vi "MB_TCP_70H16_p.vi"(6 "N":i32, 9 "timeouts":T1={"conn_timeout"=1000, "reconn_timeout"=3000, "N attempt max"=3, "t_reset_TTL"=120000, "write_timeout"=10, "read_timeout"=500, "period"=100} {"t_reset_TTL" min=10 max=240000 step=1; "period" min=10 max=100000 step=1; "read_timeout" min=10 max=60000 step=1; "write_timeout" min=1 max=60000 step=1; "N attempt max" min=1 max=5 step=1; "reconn_timeout" min=10 max=240000 step=1; "conn_timeout" min=10 max=240000}, 10 "write enable":bool=TRUE, 11 "stop":bool) -> (0 "error out":errorcluster, 2 "errors":u32, 3 "Z3":u32)   [LabVIEW 2019]
uses:
  NI_modbus_upd/NI_modbus_upd.lvlib
  NI_modbus_upd.llb/MB Modbus Command.ctl
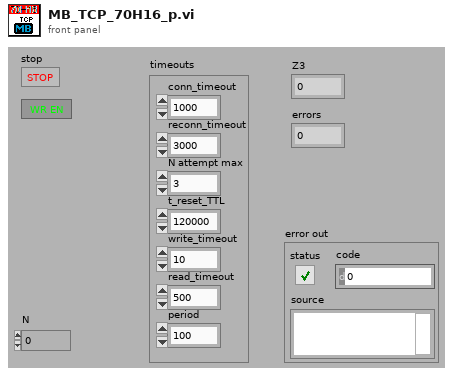
[diagram p1: front panel]
types:
  T1 = cluster{"conn_timeout":i32, "reconn_timeout":u32, "N attempt max":i32, "t_reset_TTL":u32, "write_timeout":i32, "read_timeout":i32, "period":u32}
  T2 = enum16{"Init", "Read", "Read inputs", "Read outputs", "Write", "Write inputs"}
  T3 = enum16{"DI", "DO to write", "DO", "AI", "AO to write", "AO", "DI AI", "DI AO", "DO AI", "DO AO"}
  T4 = enum16{"Start", "Connect", "Write enable", "IP address", "Errors"}
  T5 = typedef "MB Modbus Command.ctl" = cluster{"Function Code":u8, "Starting Address":u16, "Quantity":u16, "Data":u16[], "Discrete":bool[]}
  T6 = cluster{"Transaction ID":u16, "Protocol ID":u16, "Length":u16, "Unit ID":u8}
  T7 = cluster{"Remote IP Address":string, "Remote Port":u16}
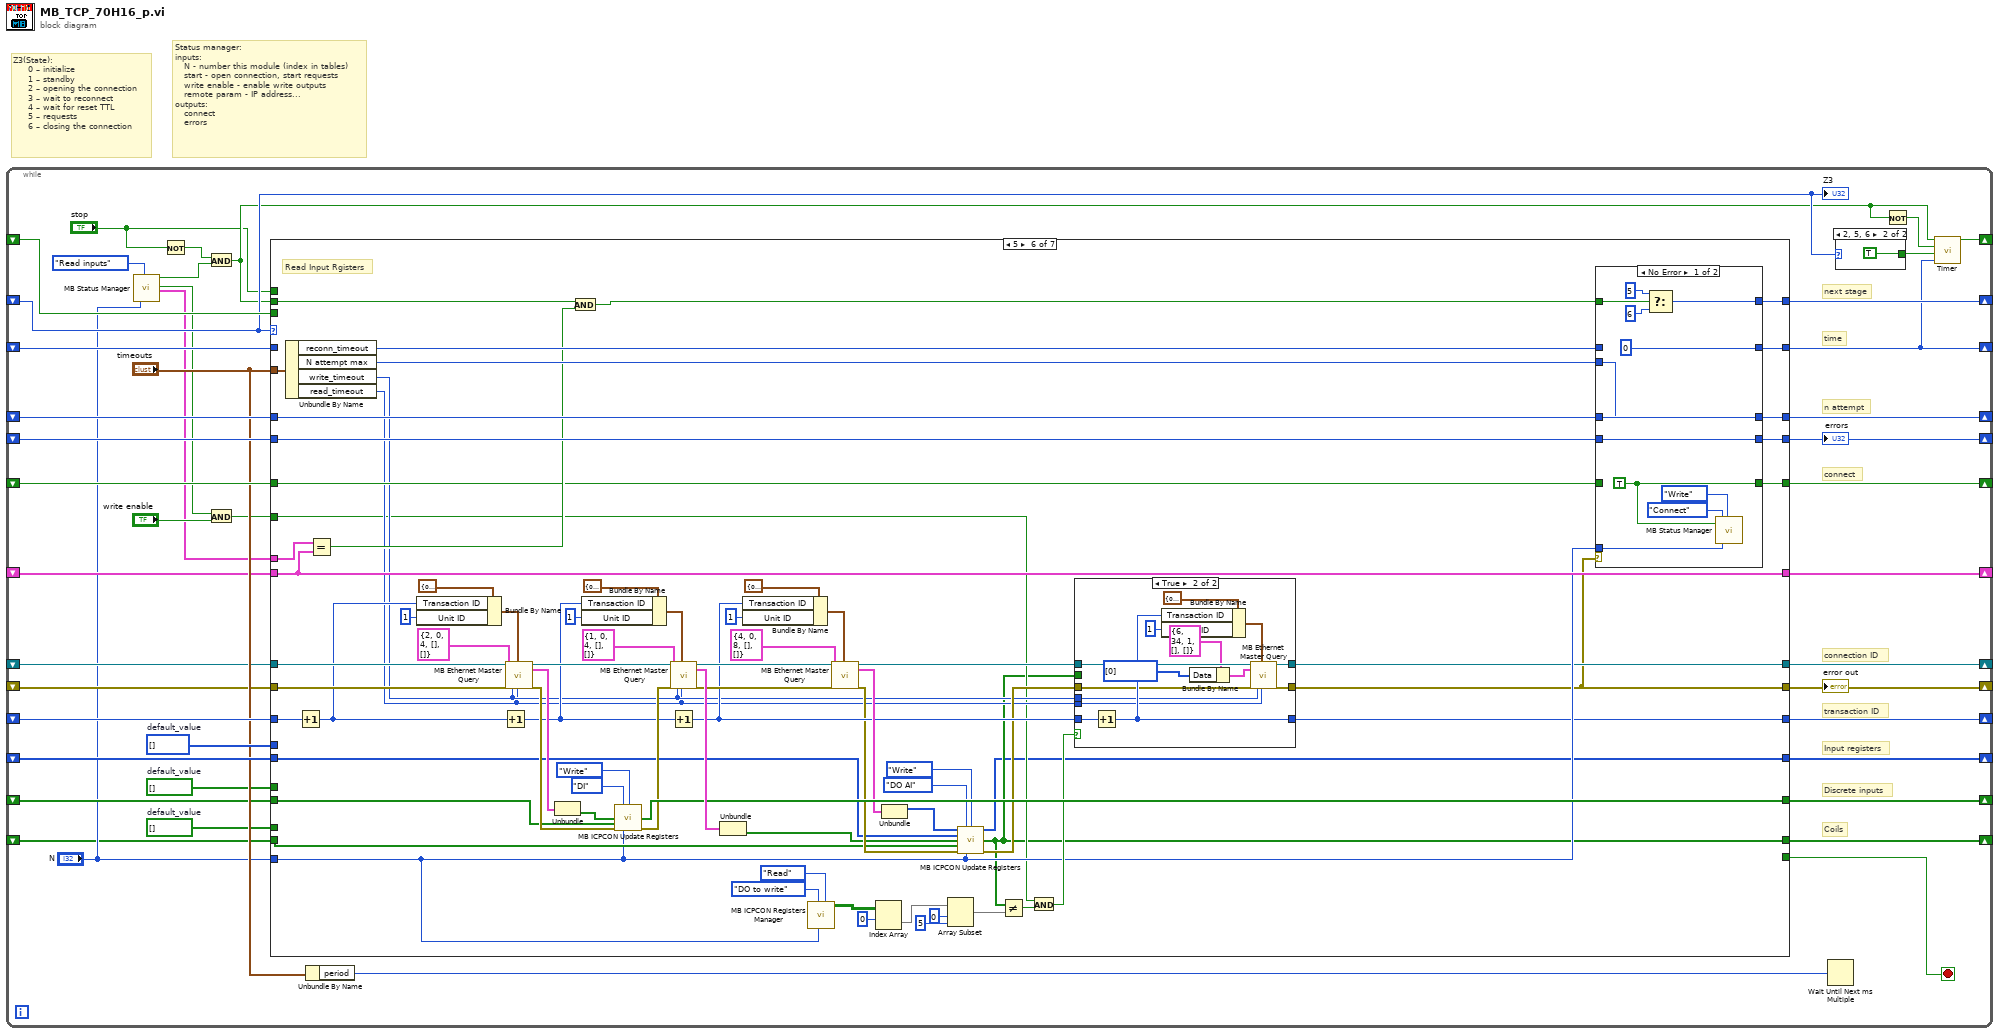
[diagram p0: block diagram]
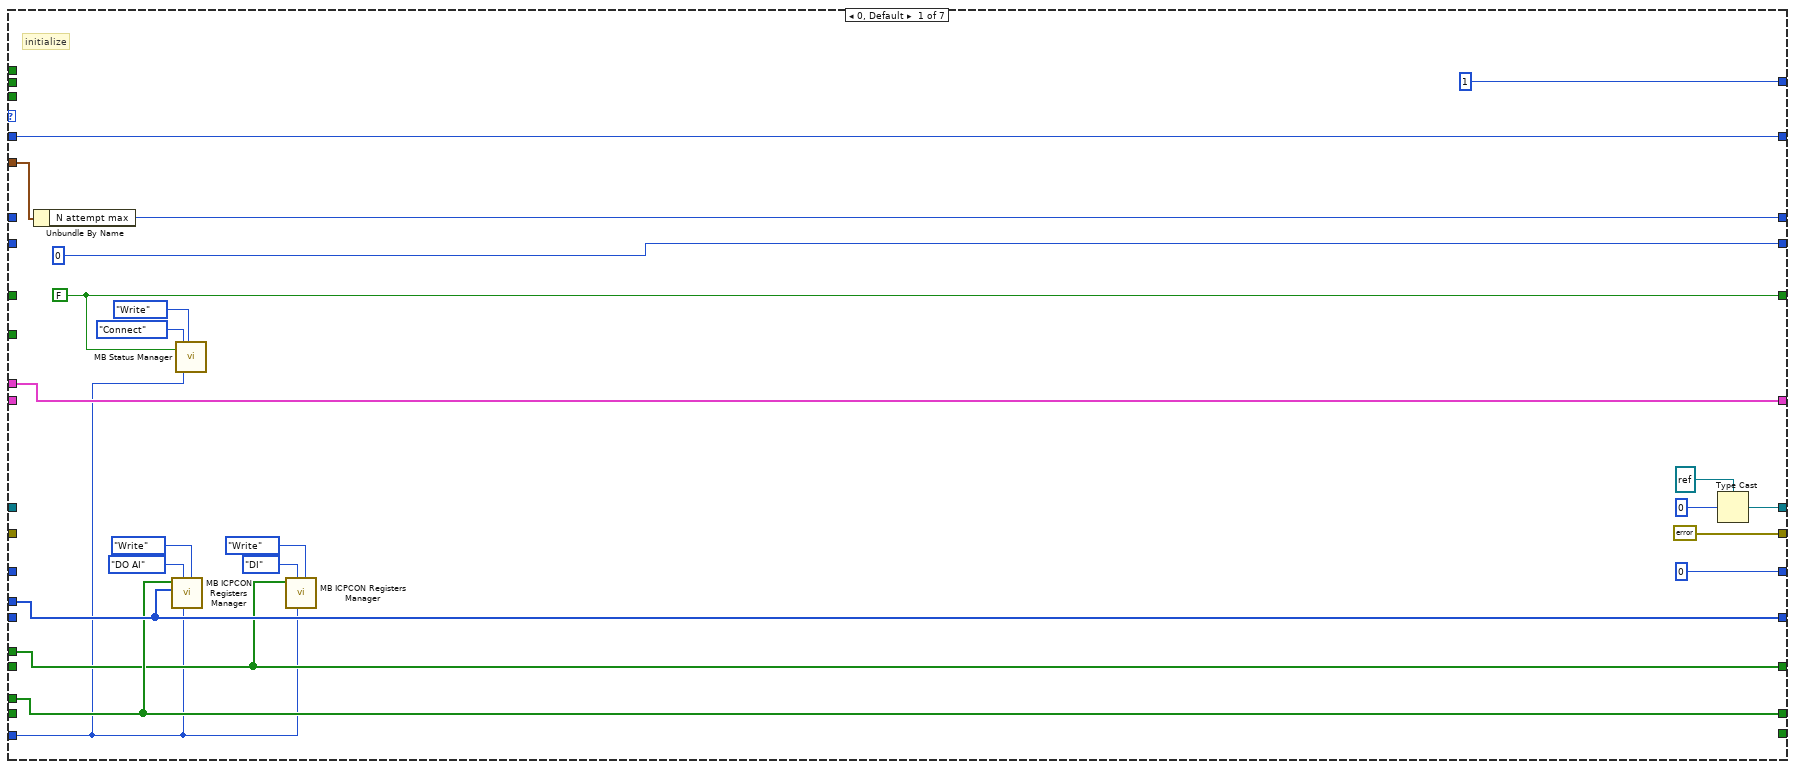
[diagram p2: hidden frame]
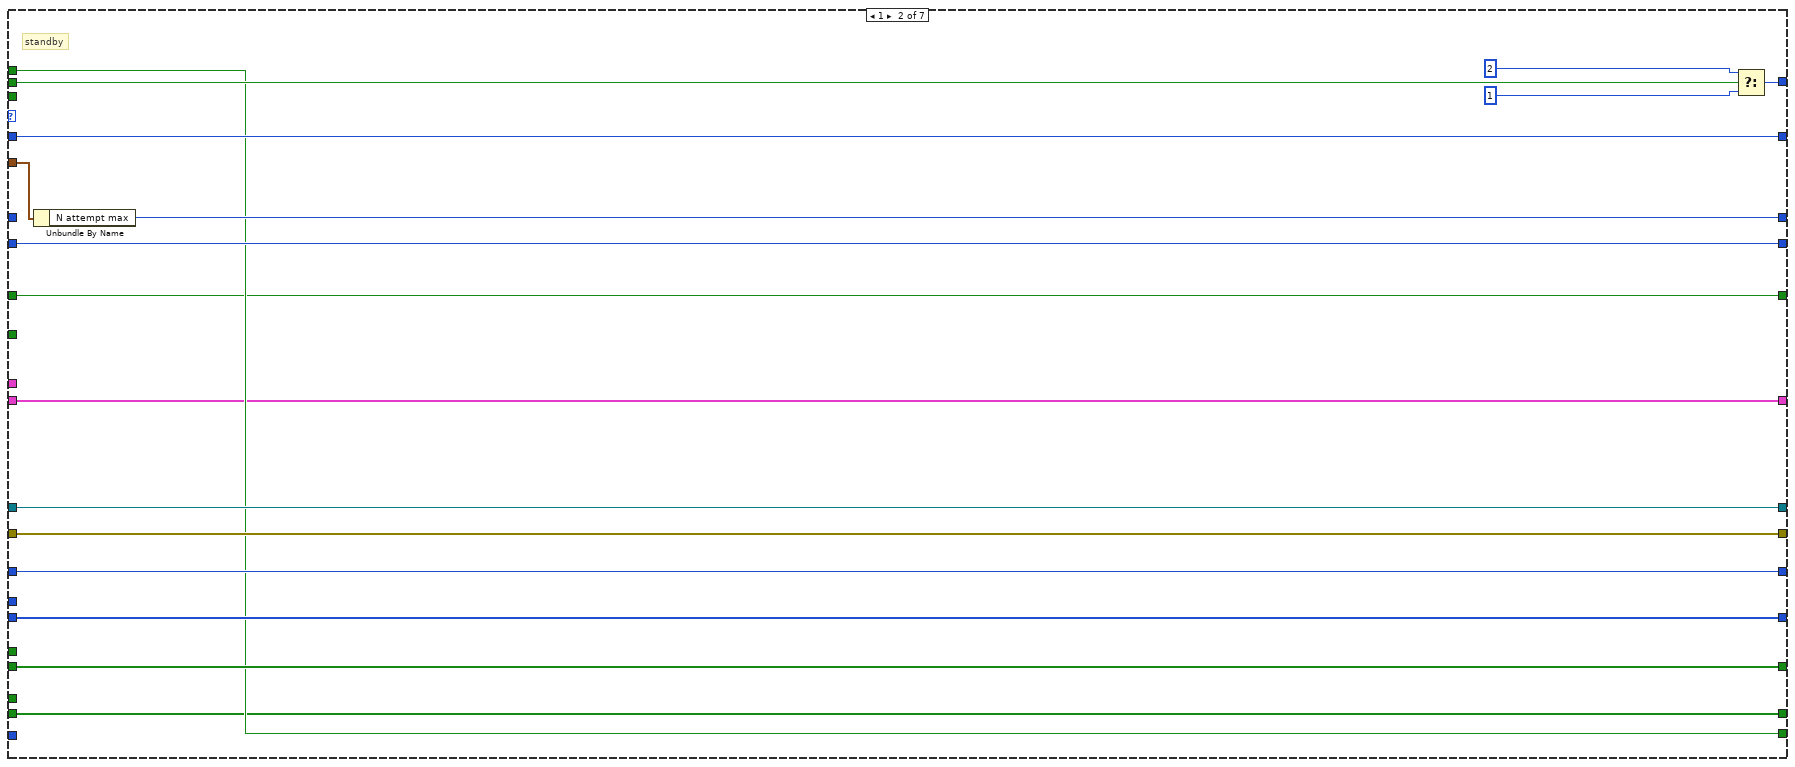
[diagram p3: hidden frame]
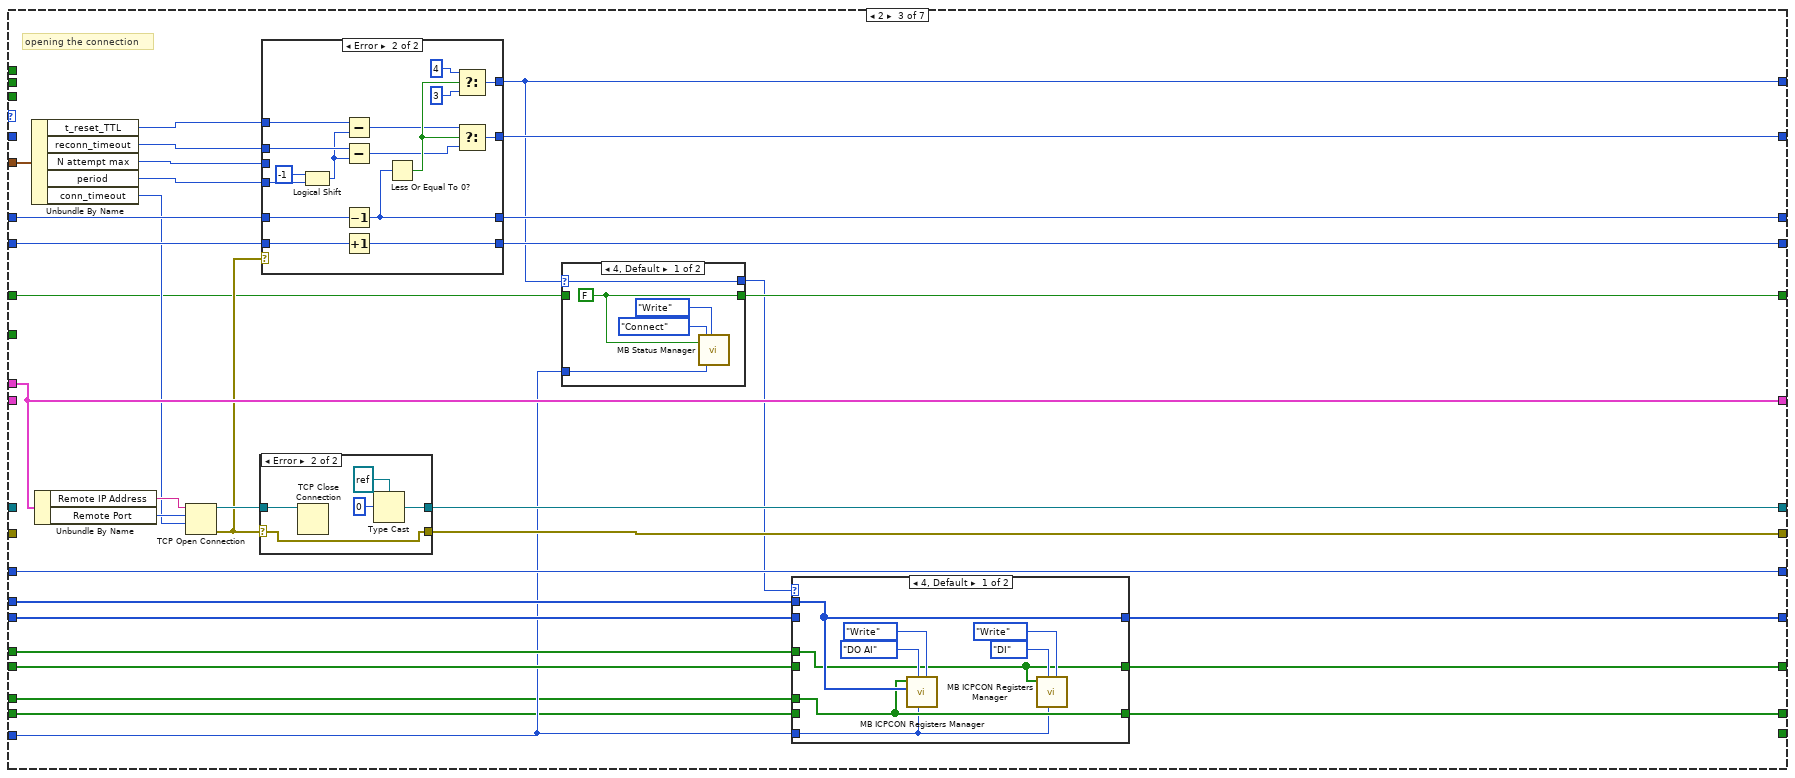
[diagram p4: hidden frame]
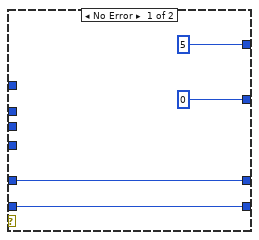
[diagram p8: hidden frame]
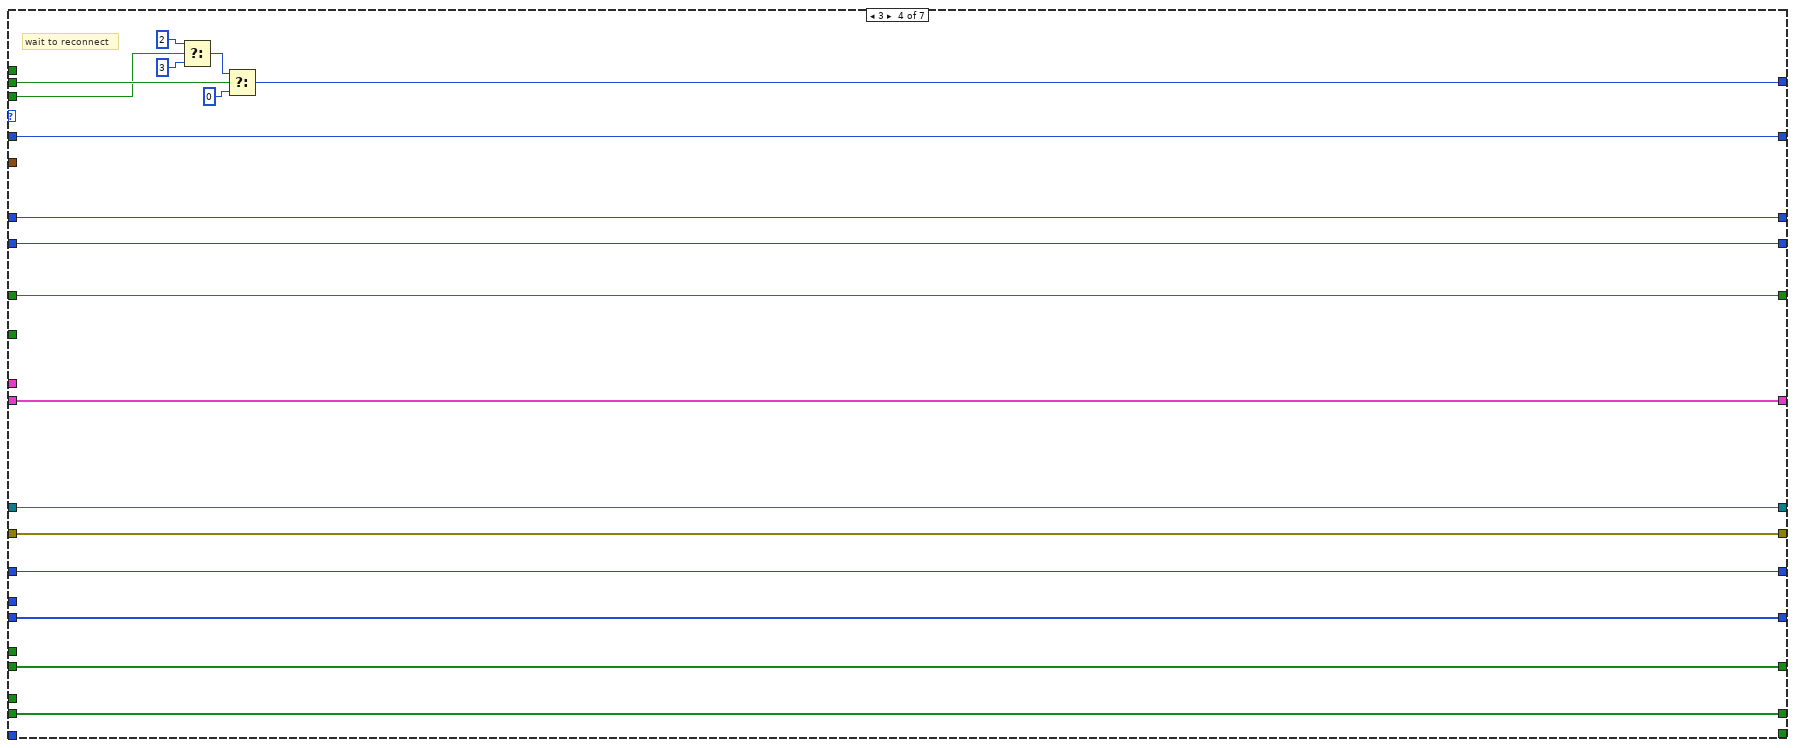
[diagram p9: hidden frame]
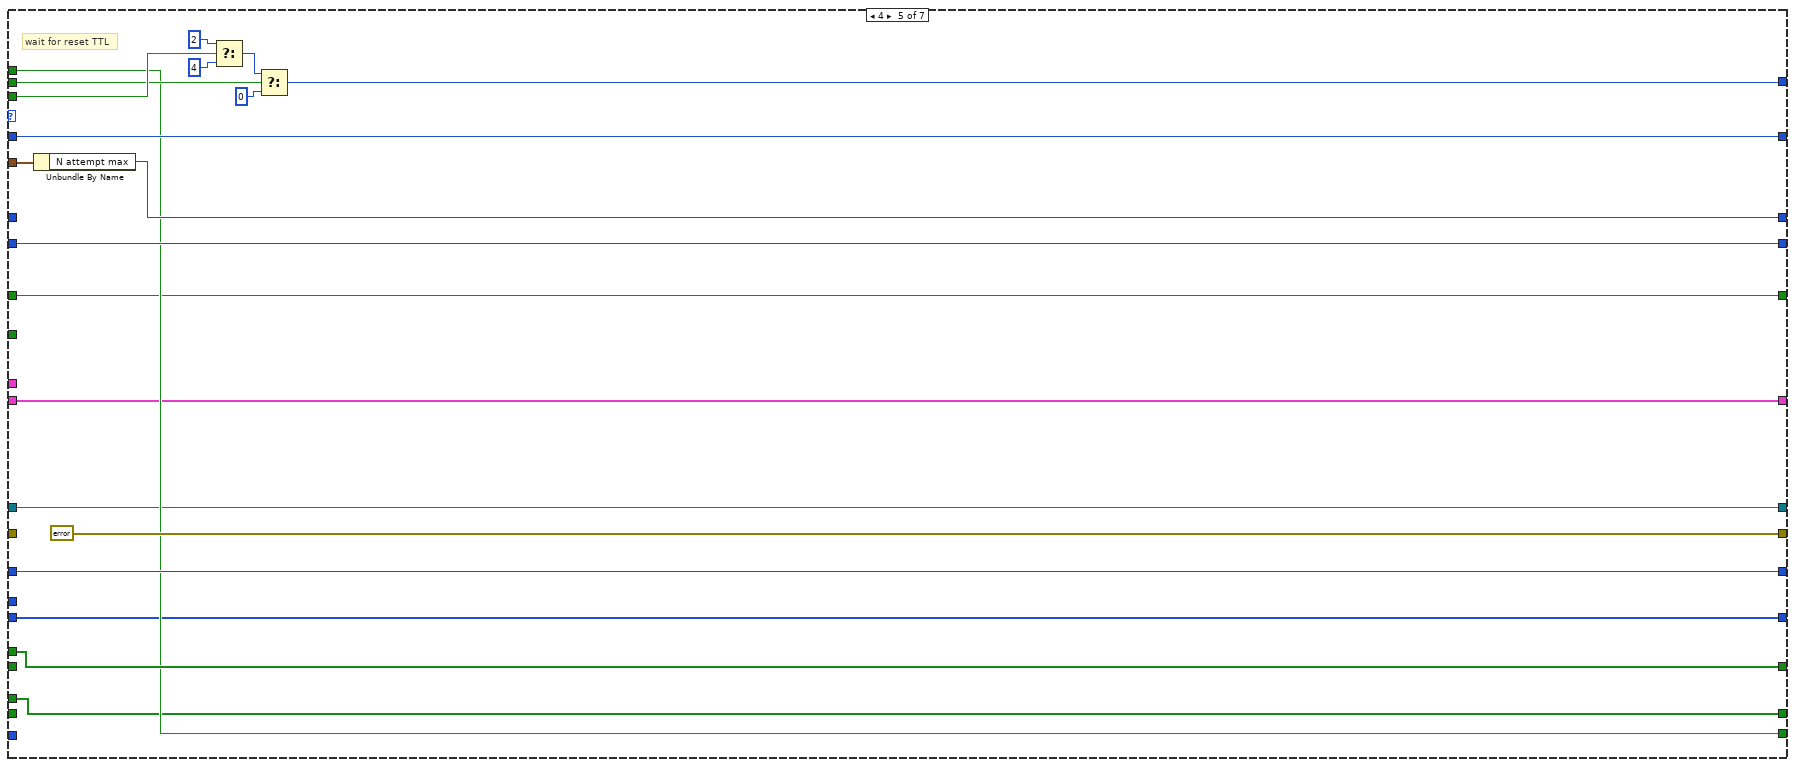
[diagram p10: hidden frame]
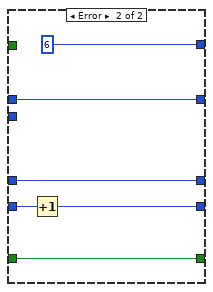
[diagram p12: hidden frame]
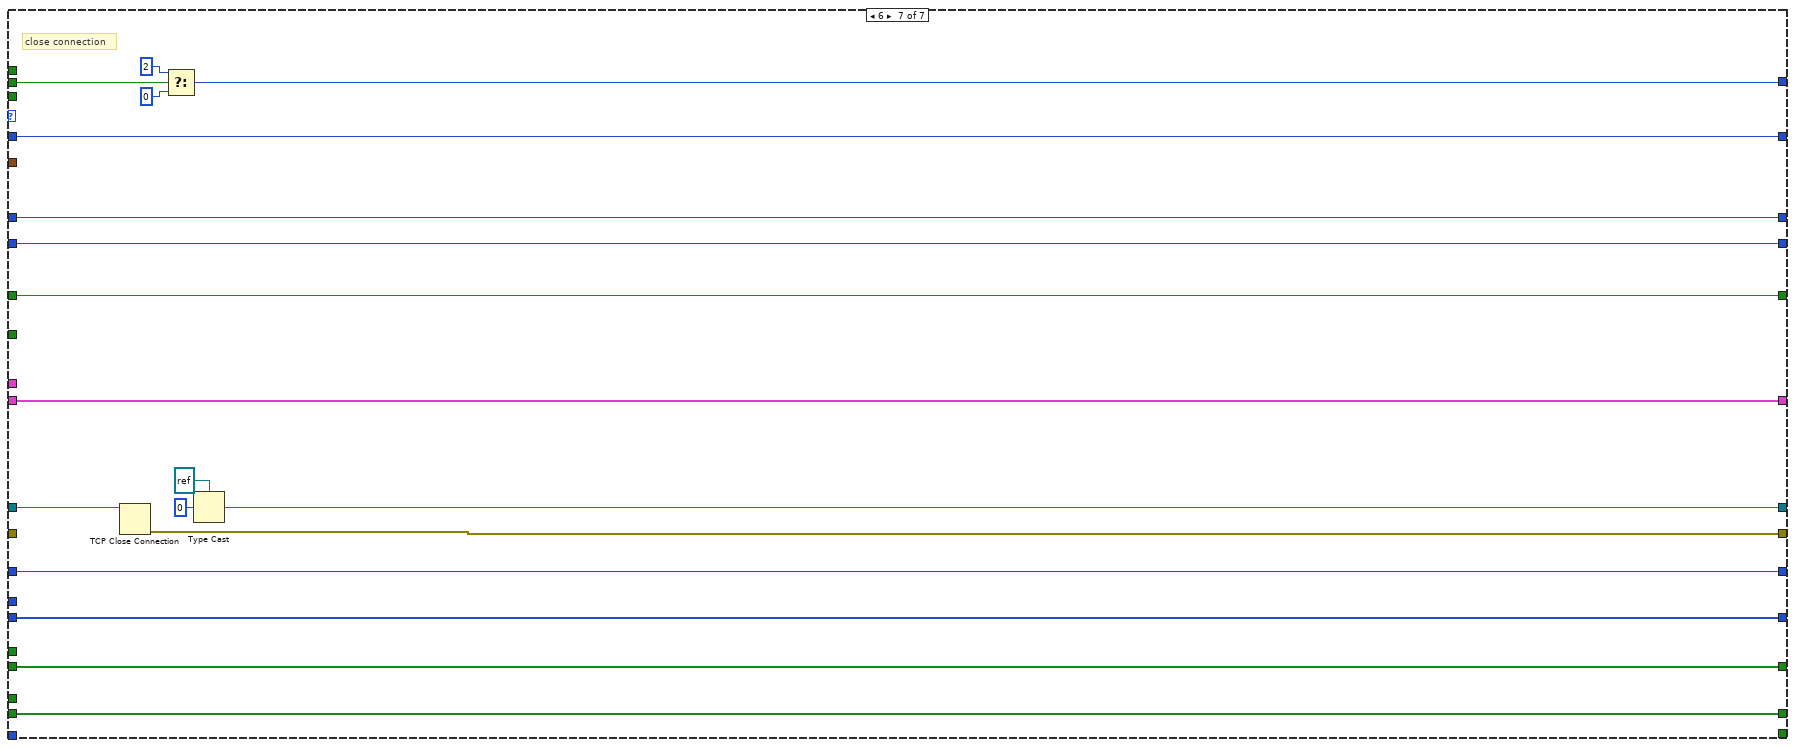
[diagram p13: hidden frame]
diagram:
  # "Status manager:\ninputs:\n   N - number this module (index in tables)\n   start - open connection, start requests\n   write enable - enable write outputs\n   remote param - IP address...\noutputs:\n   connect\n   errors"
  # "Z3(State):\n     0 – initialize \n     1 – standby\n     2 – opening the connection\n     3 – wait to reconnect\n     4 – wait for reset TTL\n     5 – requests\n     6 – closing the connection"
  n1 = while {
    shift-right: [w21] -> _
    shift-left: _ -> [w17]
    shift-right: [w20] -> _
    shift-left: _ -> [w43]
    shift-right: [w42] -> _
    shift-left: _ -> [w40]
    shift-right: [w41] -> _
    shift-left: _ -> [w39]
    shift-right: [w38] -> _
    shift-left: _ -> [w37]
    shift-right: [w36] -> _
    shift-left: _ -> [w22]
    shift-right: [w35] -> _
    shift-left: _ -> [w23]
    shift-right: [w34] -> _
    shift-left: _ -> [w33]
    shift-right: [w32] -> _
    shift-left: _ -> [w31]
    shift-right: [w25] -> _
    shift-left: _ -> [w24]
    shift-right: [w19] -> _
    shift-left: _ -> [w18]
    shift-right: [w10] -> _
    shift-left: _ -> [w9]
    shift-right: [w2] -> _
    shift-left: _ -> [w4]
    stop <- w13 stop-if-true
    w3 = bool[] []  # default_value
    w26 = bool[] []  # default_value
    w30 = u16[] []  # default_value
    # "Coils"
    # "Discrete inputs"
    # "Input registers"
    # "connect"
    # "connection ID"
    # "transaction ID"
    # "n attempt"
    # "time"
    # "next stage"
    n2 = call "MB Status Manager.vi"("N"="N", "Function"=T2."Read inputs") -> ("start"=w8:bool, "write enable"=w7:bool, "Remote Param"=w6:T7)  [unwired: 12 in, 3 out]
    n3 = Not(x="stop") -> (.not. x?=w15:bool)
    n4 = And(x=w15, y=w8) -> (x .and. y?=w16:bool)
    n5 = And(x=w7, y="write enable") -> (x .and. y?=w12:bool)
    n6 = case shown="5" w17 {
      tunnel: [w64 w74 w94 w177 w184 w201 w323] -> w36
      tunnel: [errorcluster {"status"=FALSE, "code"=0, "source"=""} ("error out") w73 w92 w176 errorcluster {"status"=FALSE, "code"=0, "source"=""} ("error out") w200 w324] -> w35
      tunnel: w22 -> [_ w74 _ w177 w184 w264 w320]
      tunnel: w23 -> [_ w73 _ w176 _ w263 _]
      tunnel: [w53 w69 w90 w165 w183 w251 w311] -> w38
      tunnel: w37 -> [_ w69 w91 w165 w183 w252 w311]
      tunnel: w6 -> [w56 _ w97 _ _ w258 _]
      tunnel: [w52 w75 w102 w164 w182 w203 w310] -> w32
      tunnel: w31 -> [_ w75 w103 w164 w182 w212 w310]
      tunnel: w33 -> [_ w83 w116 w179 w199 w273 w325]
      tunnel: [u16 0 ("x") w83 w116 w179 w199 w202 w325] -> w34
      tunnel: [w58 w79 w111 w178 w195 w271 w317] -> w42
      tunnel: w40 -> [_ _ w112 w178 _ w271 w317]
      tunnel: [u32 0 ("N attempt max") w82 w114 w175 w198 w270 w322] -> w41
      tunnel: w39 -> [_ w82 w115 w175 w198 w269 w322]
      tunnel: [w60 w81 w108 w174 w197 w266 w321] -> w20
      tunnel: w43 -> [w60 w81 _ w174 w197 _ w321]
      tunnel: "timeouts" -> [w59 w80 w113 _ w196 w272 _]
      tunnel: w16 -> [_ w71 _ w170 w186 w257 w318]
      tunnel: [u32 1 w76 w88 w166 w190 w265 w312] -> w21
      tunnel: w18 -> [_ _ _ w168 w189 _ _]
      tunnel: w30 -> [w52 _ w101 _ _ _ _]
      tunnel: w26 -> [w47 _ w98 _ w187 _ _]
      tunnel: [w47 w72 w99 w167 w187 w241 w315] -> w25
      tunnel: w24 -> [_ w72 w100 w167 _ w214 w315]
      tunnel: "N" -> [w46 _ w89 _ _ w209 _]
      tunnel: "stop" -> [_ w70 _ _ w185 _ _]
      tunnel: [_ w70 _ _ w185 _ _] -> w13
      tunnel: w12 -> [_ _ _ _ _ w205 _]
      tunnel: [w56 w68 w97 w163 w181 w255 w309] -> w10
      tunnel: w9 -> [_ w68 _ w163 w181 w255 w309]
      tunnel: w3 -> [w50 _ w86 _ w180 _ _]
      tunnel: w4 -> [_ w67 w85 w162 _ w210 w308]
      tunnel: [w50 w67 w84 w162 w180 w204 w308] -> w2
      frame 0, Default {
        w53 = FALSE ("connect")
        # "initialize"
        n7 = Unbundle By Name(w59) -> ("N attempt max"=w58:i32)
        n8 = call "MB ICPCON Registers Manager.vi"("Function"=enum16{"Init", "Read", "Write", "Read All"}."Write", "N"=w46, "Table"=T3."DO AI", "Registers In"=w52, "Discrete in"=w50) -> ()  [unwired: 4 in, 3 out]
        n9 = call "MB Status Manager.vi"("connect in"=w53, "Table"=T4."Connect", "N"=w46, "Function"=T2."Write") -> ()  [unwired: 10 in, 6 out]
        n10 = call "MB ICPCON Registers Manager.vi"("Function"=enum16{"Init", "Read", "Write", "Read All"}."Write", "N"=w46, "Table"=T3."DI", "Discrete in"=w47) -> ()  [unwired: 5 in, 3 out]
        n11 = Type Cast(type=refnum<k5> refnum ("connection ID"), x=u32 0) -> (*(type *) &x=w64:refnum<k5>)
      }
      frame 1 {
        # "standby"
        n12 = Unbundle By Name(w80) -> ("N attempt max"=w79:i32)
        n13 = Select(t=u32 2, s=w71, f=u32 1) -> (s? t:f=w76:u32)
      }
      frame 2 {
        # "opening the connection"
        n14 = Unbundle By Name(w113) -> ("t_reset_TTL"=w107:u32, "reconn_timeout"=w109:u32, "N attempt max"=w110:i32, "period"=w104:u32, "conn_timeout"=w96:i32)
        n15 = Unbundle By Name(w97) -> ("Remote IP Address"=w106:string, "Remote Port"=w105:u16)
        n16 = TCP Open Connection(address=w106, remote port or service name=w105, timeout ms (60000)=w96) -> (connection ID=w95:refnum<k5>, error out=w93:errorcluster)  [unwired: 2 in]
        n17 = case shown="Error" w93 {
          selector: w93 -> [w124 w126]
          tunnel: w95 -> [w125 w129]
          tunnel: [w125 w128] -> w94
          tunnel: [w124 w126] -> w92
          frame No Error {
          }
          frame Error {
            n18 = TCP Close Connection(connection ID=w129) -> ()  [unwired: 2 in, 2 out]
            n19 = Type Cast(type=refnum<k5> refnum ("connection ID"), x=u32 0) -> (*(type *) &x=w128:refnum<k5>)
          }
        }
        n20 = case shown="Error" w93 {
          tunnel: w115 -> [w145 w161]
          tunnel: [w145 w160] -> w114
          tunnel: w112 -> [w144 w159]
          tunnel: [w144 w158] -> w111
          tunnel: w110 -> [_ _]
          tunnel: [u32 5 w155] -> w88
          tunnel: w109 -> [_ w154]
          tunnel: [u32 0 w153] -> w108
          tunnel: w107 -> [_ w150]
          tunnel: w104 -> [_ w148]
          frame No Error {
          }
          frame Error {
            n21 = Logical Shift(y=i16 -1, x=w148) -> (x << y=w146:u32)
            n22 = Subtract(x=w150, y=w146) -> (x-y=w149:u32)
            n23 = Subtract(x=w154, y=w146) -> (x-y=w151:u32)
            n24 = Decrement(x=w159) -> (x-1=w158:i32)
            n25 = Increment(x=w161) -> (x+1=w160:u32)
            n26 = Less Or Equal To 0?(x=w158) -> (x <= 0?=w152:bool)
            n27 = Select(t=u32 4, s=w152, f=u32 3) -> (s? t:f=w155:u32)
            n28 = Select(t=w149, s=w152, f=w151) -> (s? t:f=w153:u32)
          }
        }
        n29 = case shown="4, Default" w88 {
          selector: w88 -> [w118 w122]
          tunnel: w89 -> [w119 _]
          tunnel: [w120 w123] -> w90
          tunnel: w91 -> [_ w123]
          tunnel: [w118 w122] -> w87
          frame 4, Default {
            w120 = FALSE ("f")
            n30 = call "MB Status Manager.vi"("connect in"=w120, "Table"=T4."Connect", "N"=w119, "Function"=T2."Write") -> ()  [unwired: 10 in, 6 out]
          }
          frame 3, 5 {
          }
        }
        n31 = case shown="4, Default" w87 {
          tunnel: w89 -> [w132 _]
          tunnel: [w136 w141] -> w102
          tunnel: w103 -> [_ w141]
          tunnel: w101 -> [w136 _]
          tunnel: w100 -> [_ w140]
          tunnel: [w131 w140] -> w99
          tunnel: w98 -> [w131 _]
          tunnel: w86 -> [w135 _]
          tunnel: [w135 w139] -> w84
          tunnel: w85 -> [_ w139]
          frame 4, Default {
            n32 = call "MB ICPCON Registers Manager.vi"("Function"=enum16{"Init", "Read", "Write", "Read All"}."Write", "N"=w132, "Table"=T3."DO AI", "Registers In"=w136, "Discrete in"=w135) -> ()  [unwired: 4 in, 3 out]
            n33 = call "MB ICPCON Registers Manager.vi"("Function"=enum16{"Init", "Read", "Write", "Read All"}."Write", "N"=w132, "Table"=T3."DI", "Discrete in"=w131) -> ()  [unwired: 5 in, 3 out]
          }
          frame 3, 5 {
          }
        }
      }
      frame 3 {
        # "wait to reconnect"
        n34 = Select(t=u32 2, s=w168, f=u32 3) -> (s? t:f=w169:u32)
        n35 = Select(t=w169, s=w170, f=u32 0) -> (s? t:f=w166:u32)
      }
      frame 4 {
        # "wait for reset TTL"
        n36 = Unbundle By Name(w196) -> ("N attempt max"=w195:i32)
        n37 = Select(t=u32 2, s=w189, f=u32 4) -> (s? t:f=w191:u32)
        n38 = Select(t=w191, s=w186, f=u32 0) -> (s? t:f=w190:u32)
      }
      frame 5 {
        # "Read Input Rgisters"
        n39 = Unbundle By Name(w272) -> ("reconn_timeout"=w267:u32, "N attempt max"=w268:i32, "write_timeout"=w207:i32, "read_timeout"=w206:i32)
        n40 = Increment(x=w273) -> (x+1=w245:u16)
        n41 = Equal?(x=w258, y=w255) -> (x = y?=w254:bool)
        n42 = Bundle By Name(cluster=T6 {"Transaction ID"=0, "Protocol ID"=0, "Length"=0, "Unit ID"=0} ("MBAP Header"), "Transaction ID"=w245, "Unit ID"=u8 1) -> (w259:T6)
        n43 = Increment(x=w245) -> (x+1=w229:u16)
        n44 = call "MB Ethernet Master Query.vi"("TCP Connection Refnum in"=w264, "Modbus Command"=T5 {"Function Code"=2, "Starting Address"=0, "Quantity"=4, "Data"=[], "Discrete"=[]}, "error in (no error)"=w263, "Write Timeout"=w207, "MBAP Header"=w259, "Read Timeout"=w206) -> ("TCP Connection Refnum (dup)"=w239:refnum<k5>, "Registers"=w262:cluster{"Registers":u16[], "Discrete":bool[]}, "error out"=w238:errorcluster)  [unwired: 9 in, 2 out]
        n45 = Unbundle(w262) -> ("Discrete"=w215:bool[])  [unwired: 1 out]
        n46 = And(x=w257, y=w254) -> (x .and. y?=w256:bool)
        n47 = Bundle By Name(cluster=T6 {"Transaction ID"=0, "Protocol ID"=0, "Length"=0, "Unit ID"=0} ("MBAP Header"), "Transaction ID"=w229, "Unit ID"=u8 1) -> (w248:T6)
        n48 = call "MB ICPCON Update Registers.vi"("Table"=T3."DI", "Function"=enum16{"Init", "Read", "Write", "Read All"}."Write", "Discrete in"=w215, "Default Discrete in"=w214, "error in (no error)"=w238, "N"=w209) -> ("Discretes"=w241:bool[], "error out"=w237:errorcluster)  [unwired: 7 in, 1 out]
        n49 = call "MB Ethernet Master Query.vi"("TCP Connection Refnum in"=w239, "Modbus Command"=T5 {"Function Code"=1, "Starting Address"=0, "Quantity"=4, "Data"=[], "Discrete"=[]} ("MODBUS Command"), "error in (no error)"=w237, "Write Timeout"=w207, "MBAP Header"=w248, "Read Timeout"=w206) -> ("TCP Connection Refnum (dup)"=w231:refnum<k5>, "Registers"=w243:cluster{"Registers":u16[], "Discrete":bool[]}, "error out"=w228:errorcluster)  [unwired: 9 in, 2 out]
        n50 = Increment(x=w229) -> (x+1=w227:u16)
        n51 = Unbundle(w243) -> ("Discrete"=w211:bool[])  [unwired: 1 out]
        n52 = Bundle By Name(cluster=T6 {"Transaction ID"=0, "Protocol ID"=0, "Length"=0, "Unit ID"=0} ("MBAP Header"), "Transaction ID"=w227, "Unit ID"=u8 1) -> (w232:T6)
        n53 = call "MB ICPCON Registers Manager.vi"("Function"=enum16{"Init", "Read", "Write", "Read All"}."Read", "N"=w209, "Table"=T3."DO to write") -> ("Discretes"=w222:bool[][])  [unwired: 6 in, 2 out]
        n54 = call "MB Ethernet Master Query.vi"("TCP Connection Refnum in"=w231, "Modbus Command"=T5 {"Function Code"=4, "Starting Address"=0, "Quantity"=8, "Data"=[], "Discrete"=[]} ("MODBUS Command"), "error in (no error)"=w228, "MBAP Header"=w232) -> ("TCP Connection Refnum (dup)"=w230:refnum<k5>, "Registers"=w236:cluster{"Registers":u16[], "Discrete":bool[]}, "error out"=w217:errorcluster)  [unwired: 11 in, 2 out]
        n55 = Index Array(array=w222, index (row)=0) -> (element=w220:bool[])  [unwired: 1 in]
        n56 = Unbundle(w236) -> ("Registers"=w213:u16[])  [unwired: 1 out]
        n57 = Array Subset(array=w220, index=0, length=5) -> (w208:bool[])
        n58 = call "MB ICPCON Update Registers.vi"("Registers In"=w213, "Table"=T3."DO AI", "Function"=enum16{"Init", "Read", "Write", "Read All"}."Write", "Default Registers In"=w212, "Discrete in"=w211, "Default Discrete in"=w210, "error in (no error)"=w217, "N"=w209) -> ("Registers"=w203:u16[], "Discretes"=w204:bool[], "error out"=w216:errorcluster)  [unwired: 5 in]
        n59 = Not Equal?(x=w204, y=w208) -> (x != y?=w242:bool)
        n60 = And(x=w205, y=w242) -> (x .and. y?=w240:bool)
        n61 = case shown="True" w240 {
          tunnel: w206 -> [_ w281]
          tunnel: w207 -> [_ w280]
          tunnel: w227 -> [w275 w288]
          tunnel: [w275 w287] -> w202
          tunnel: w216 -> [w274 w285]
          tunnel: [w274 w284] -> w200
          tunnel: w230 -> [w276 w283]
          tunnel: [w276 w282] -> w201
          tunnel: w204 -> [_ _]
          frame False {
          }
          frame True {
            n62 = Increment(x=w288) -> (x+1=w287:u16)
            n63 = Bundle By Name(cluster=T6 {"Transaction ID"=0, "Protocol ID"=0, "Length"=0, "Unit ID"=0} ("MBAP Header"), "Transaction ID"=w287, "Unit ID"=u8 1) -> (w289:T6)
            n64 = Bundle By Name(cluster=T5 {"Function Code"=6, "Starting Address"=34, "Quantity"=1, "Data"=[], "Discrete"=[]} ("MODBUS Command"), "Data"=u16[] [0]) -> (w278:T5)
            n65 = call "MB Ethernet Master Query.vi"("TCP Connection Refnum in"=w283, "Modbus Command"=w278, "error in (no error)"=w285, "Write Timeout"=w280, "MBAP Header"=w289, "Read Timeout"=w281) -> ("TCP Connection Refnum (dup)"=w282:refnum<k5>, "error out"=w284:errorcluster)  [unwired: 9 in, 3 out]
          }
        }
        n66 = case shown="No Error" w200 {
          tunnel: w269 -> [w295 w307]
          tunnel: [w295 w306] -> w270
          tunnel: [w297 u32 6] -> w265
          tunnel: w271 -> [_ w304]
          tunnel: w268 -> [w301 _]
          tunnel: [w301 w304] -> _
          tunnel: w267 -> [_ w303]
          tunnel: [u32 0 w303] -> w266
          tunnel: w256 -> [w296 _]
          tunnel: w252 -> [_ w302]
          tunnel: [w293 w302] -> w251
          tunnel: w209 -> [w292 _]
          frame No Error {
            w293 = TRUE ("f")
            n67 = Select(t=u32 5, s=w296, f=u32 6) -> (s? t:f=w297:u32)
            n68 = call "MB Status Manager.vi"("connect in"=w293, "Table"=T4."Connect", "N"=w292, "Function"=T2."Write") -> ()  [unwired: 10 in, 6 out]
          }
          frame Error {
            n69 = Increment(x=w307) -> (x+1=w306:u32)
          }
        }
      }
      frame 6 {
        # "close connection"
        n70 = TCP Close Connection(connection ID=w320) -> (error out=w324:errorcluster)  [unwired: 2 in, 1 out]
        n71 = Select(t=u32 2, s=w318, f=u32 0) -> (s? t:f=w312:u32)
        n72 = Type Cast(type=refnum<k5> refnum ("connection ID"), x=u32 0) -> (*(type *) &x=w323:refnum<k5>)
      }
    }
    "error out" <- w35
    "errors" <- w41
    n73 = Unbundle By Name("timeouts") -> ("period"=w28:u32)
    n74 = Wait Until Next ms Multiple(millisecond multiple=w28) -> ()  [unwired: 1 out]
    n75 = case shown="2, 5, 6" w17 {
      tunnel: [_ TRUE] -> w27
      frame 0, Default {
      }
      frame 2, 5, 6 {
      }
    }
    n76 = Not(x=w16) -> (.not. x?=w44:bool)
    n77 = call "Timer.vi"("ms"=w20, "Load (F)"=w27, "Reset (F)"=w44, "Start (T)"=w16) -> ("End"=w19:bool)  [unwired: 5 in, 1 out]
    "Z3" <- w17
  }
